vi "runNextScript.vi"(5 "Loop?":bool=TRUE, 6 "keepRunning in":bool, 7 "Increment Script Number?":bool, 8 "error in (no error)":errorcluster, 9 "Listbox in":refnum<vi>, 10 "status in":refnum<vi>, 11 "ExperimentRunner in":refnum<class "ExperimentRunner.lvclass">) -> (0 "error out":errorcluster, 1 "Listbox out":refnum<vi>, 2 "status out":refnum<vi>, 3 "ExperimentRunner out":refnum<class "ExperimentRunner.lvclass">, 4 "keepRunning":bool)   [LabVIEW 2009, in "Views.lvlib" / "ExperimentControl.lvlib" / "ExperimentRunner.lvclass"]
uses:
  ExperimentRunner.lvclass
  ExperimentRunner.lvclass/ExperimentRunner.ctl
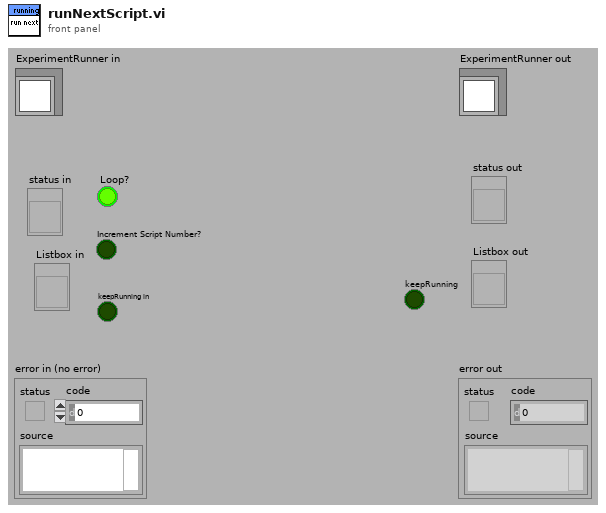
[diagram p1: front panel]
types:
  T1 = enum16{"Ready", "Compiling", "Configured", "Running", "Stopping", "Unresolved Error"}
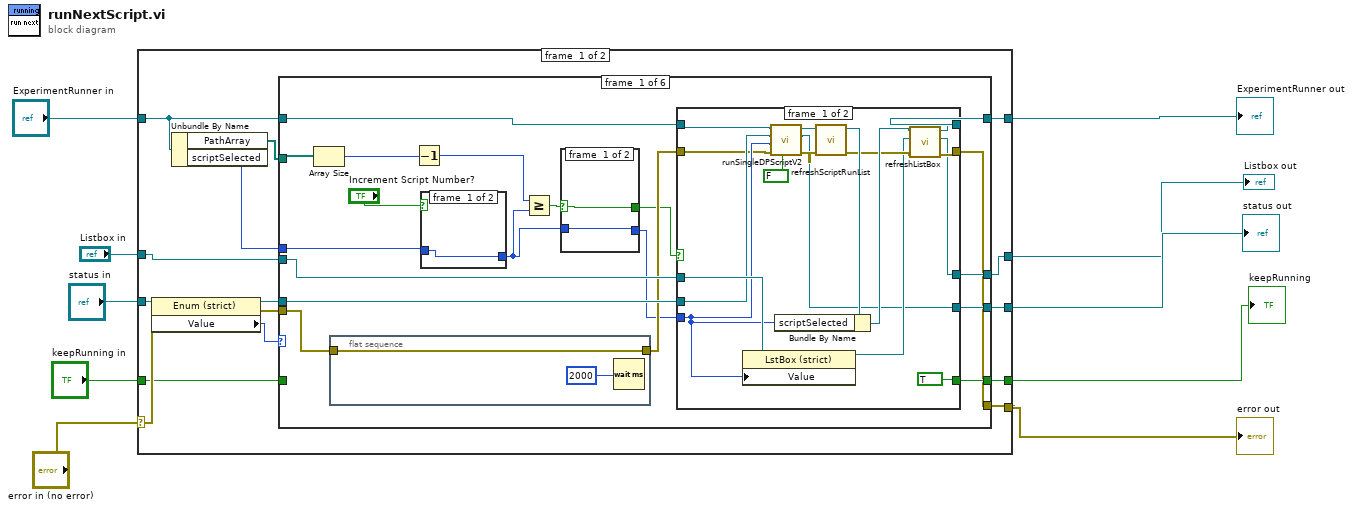
[diagram p0: block diagram]
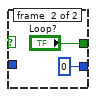
[diagram p2: hidden frame]
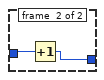
[diagram p3: hidden frame]
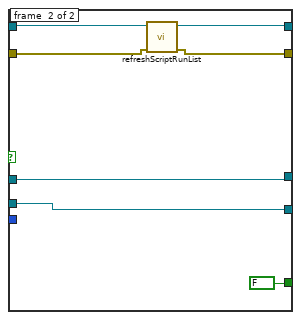
[diagram p4: hidden frame]
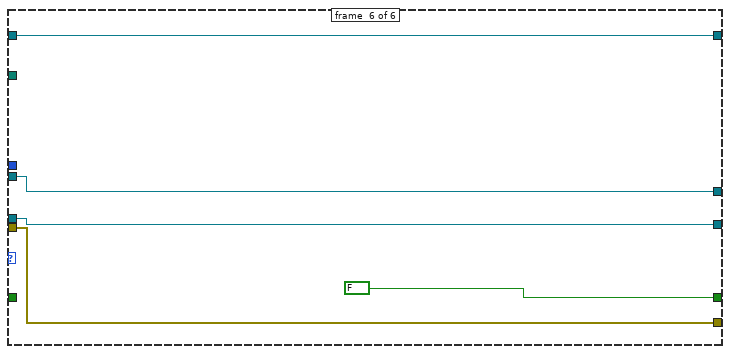
[diagram p9: hidden frame]
diagram:
  n1 = case shown="No Error" "error in (no error)" {
    selector: "error in (no error)" -> [w21 w104]
    tunnel: [w12 w104] -> w9
    tunnel: [w17 w103] -> w7
    tunnel: "ExperimentRunner in" -> [w20 w103]
    tunnel: "status in" -> [w25 _]
    tunnel: [w11 _] -> w5
    tunnel: "keepRunning in" -> [w19 _]
    tunnel: [w15 _] -> w3
    tunnel: "Listbox in" -> [w14 _]
    tunnel: [w13 _] -> w1
    frame #0 {
      n2 = property class="Enum (strict)"(reference=w25, error in=w21) -> (reference out=w23:refnum<vi>, error out=w22:errorcluster, "Value"=w24:T1)
      n3 = Unbundle By Name(w20) -> ("PathArray"=w16:path[], "scriptSelected"=w18:i32)
      n4 = case shown="\"Ready\", Default" w24 {
        tunnel: w23 -> [w39 w80 w84 w90 w96 w99]
        tunnel: w22 -> [w34 w79 w83 w88 w95 w98]
        tunnel: w20 -> [w41 w82 w86 w91 w94 w101]
        tunnel: [w40 w78 w87 w92 w93 FALSE] -> w11
        tunnel: w19 -> [_ w78 w87 w92 w93 _]
        tunnel: w18 -> [w32 _ _ _ _ _]
        tunnel: [w42 w82 w86 w91 w94 w101] -> w17
        tunnel: w16 -> [w44 _ _ _ _ _]
        tunnel: [w38 w80 w84 w90 w96 w99] -> w15
        tunnel: w14 -> [w37 w81 w85 w89 w97 w100]
        tunnel: [w36 w81 w85 w89 w97 w100] -> w13
        tunnel: [w35 w79 w83 w88 w95 w98] -> w12
        frame #0 {
          n5 = Array Size(array=w44) -> (size(s)=w43:i32)
          n6 = flat-sequence {
            tunnel: w34 -> [w52]
            tunnel: [w52] -> w33
            frame #0 {
              n7 = Wait (ms)(milliseconds to wait=2000) -> ()  [unwired: 1 out]
            }
          }
          n8 = Decrement(x=w43) -> (x-1=w29:i32)
          n9 = case shown="True" "Increment Script Number?" {
            tunnel: w32 -> [w49 w51]
            tunnel: [w49 w50] -> w28
            frame #0 {
            }
            frame #1 {
              n10 = Increment(x=w51) -> (x+1=w50:i32)
            }
          }
          n11 = Greater Or Equal?(x=w29, y=w28) -> (x >= y?=w26:bool)
          n12 = case shown="True" w26 {
            selector: w26 -> [w45 _]
            tunnel: [w45 "Loop?"] -> w30
            tunnel: w28 -> [w46 _]
            tunnel: [w46 0 ("scriptSelected")] -> w27
            frame #0 {
            }
            frame #1 {
            }
          }
          n13 = case shown="True" w30 {
            tunnel: [w66 w71] -> w42
            tunnel: w41 -> [w61 w74]
            tunnel: [TRUE FALSE] -> w40
            tunnel: w27 -> [w56 _]
            tunnel: w39 -> [w57 w76]
            tunnel: [w58 w76] -> w38
            tunnel: w37 -> [w70 w75]
            tunnel: [w62 w75] -> w36
            tunnel: w33 -> [w55 w73]
            tunnel: [w64 w72] -> w35
            frame #0 {
              n14 = property class="LstBox (strict)"(reference=w70, "Value"=w56) -> (reference out=w63:refnum<vi>)  [unwired: 1 in, 1 out]
              n15 = call "runSingleDPScriptV2.vi"("HWLoop?"=FALSE, "error in (no error)"=w55, "index"=w56, "status in"=w57, "ExperimentRunner in"=w61) -> ("error out"=w59:errorcluster, "status out"=w58:refnum<vi>, "ExperimentRunner out"=w60:refnum<class "ExperimentRunner.lvclass">)  [unwired: 4 in]
              n16 = call "refreshScriptRunList.vi"("error in (no error)"=w59, "ExperimentRunner in"=w60) -> ("error out"=w65:errorcluster, "ExperimentRunner out"=w68:refnum<class "ExperimentRunner.lvclass">)  [unwired: 8 in]
              n17 = Bundle By Name(cluster=w68, "scriptSelected"=w56) -> (w67:refnum<class "ExperimentRunner.lvclass">)
              n18 = call "refreshListBox.vi"("error in (no error)"=w65, "Listbox"=w63, "ExperimentRunner in"=w67) -> ("error out"=w64:errorcluster, "Listbox out"=w62:refnum<vi>, "ExperimentRunner out"=w66:refnum<class "ExperimentRunner.lvclass">)  [unwired: 6 in]
            }
            frame #1 {
              n19 = call "refreshScriptRunList.vi"("error in (no error)"=w73, "ExperimentRunner in"=w74) -> ("error out"=w72:errorcluster, "ExperimentRunner out"=w71:refnum<class "ExperimentRunner.lvclass">)  [unwired: 8 in]
            }
          }
        }
        frame #1 {
        }
        frame #2 {
        }
        frame #3 {
        }
        frame #4 {
        }
        frame #5 {
        }
      }
    }
    frame #1 {
    }
  }
  "error out" <- w9
  "ExperimentRunner out" <- w7
  "status out" <- w3
  "keepRunning" <- w5
  "Listbox out" <- w1
